vi "AddLeft.vi"(11 "Array":i32[](array[numeric])=[2, 2, 4, 4]) -> (0 "score":i32, 3 "Array 2":i32[](array[numeric])=[0, 3, 2, 1], 5 "tiles moved?":bool)   [LabVIEW 2010]
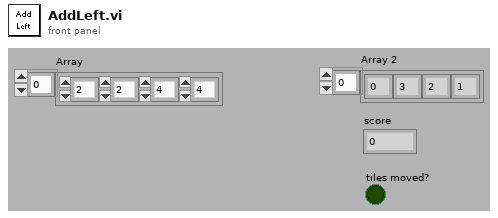
[diagram p1: front panel]
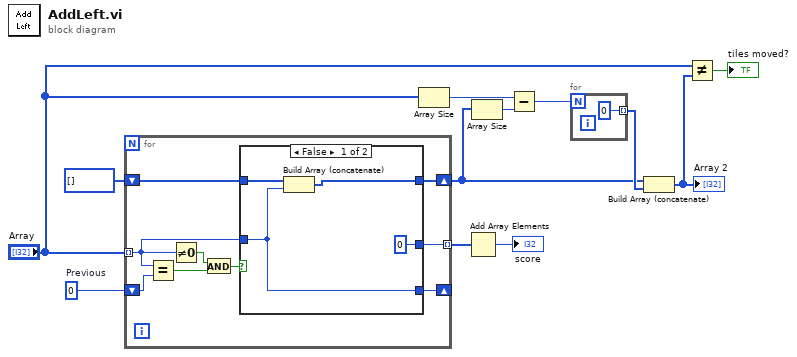
[diagram p0: block diagram]
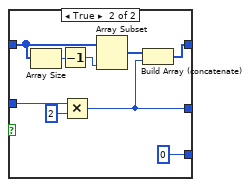
[diagram p2: hidden frame]
diagram:
  w11 = 0  # Previous
  n1 = for {
    shift-right: [w19] -> w7
    shift-left: i32[] [] ("Array") -> [w20]
    tunnel: "Array" -> [w14] mode=indexing
    shift-right: [w18] -> _
    shift-left: w11 -> [w21]
    tunnel: [w13] -> w6 mode=indexing
    n2 = Equal?(x=w14, y=w21) -> (x = y?=w17:bool)
    n3 = Not Equal To 0?(x=w14) -> (x != 0?=w15:bool)
    n4 = And(x=w15, y=w17) -> (x .and. y?=w16:bool)
    n5 = case shown="False" w16 {
      tunnel: w20 -> [w25 w28]
      tunnel: w14 -> [w23 w34]
      tunnel: [w24 w32] -> w19
      tunnel: [w23 0 ("Previous")] -> w18
      tunnel: [0 w26] -> w13
      frame False {
        n6 = Build Array (concatenate)(w25, w23) -> (w24:i32[])
      }
      frame True {
        n7 = Array Size(array=w28) -> (size(s)=w29:i32)
        n8 = Decrement(x=w29) -> (x-1=w27:i32)
        n9 = Multiply(x=w34, y=2) -> (x*y=w26:i32)
        n10 = Array Subset(array=w28, length=w27) -> (w30:i32[])  [unwired: 1 in]
        n11 = Build Array (concatenate)(w30, w26) -> (w32:i32[])
      }
    }
  }
  n12 = Array Size(array="Array") -> (size(s)=w8:i32)
  n13 = Add Array Elements(numeric array=w6) -> (sum=→"score":i32)
  n14 = Array Size(array=w7) -> (size(s)=w10:i32)
  n15 = Subtract(x=w8, y=w10) -> (x-y=w4:i32)
  n16 = for {
    N: w4 -> [_]
    tunnel: [0 ("Numeric")] -> w9 mode=indexing
  }
  n17 = Build Array (concatenate)(w7, w9) -> (w2:i32[])
  "Array 2" <- w2
  n18 = Not Equal?(x="Array", y=w2) -> (x != y?=→"tiles moved?":bool)
